vi "GeoData.vi"() -> ()   [LabVIEW 2017] (continued)
PA\tPhiladelphia County\tH6\n19124\t42101\tPhiladelphia\tPA\tPhiladelphia County\tH6\n19152\t42101\tPhiladelphia\tPA\tPhiladelphia County\tH6\n19110\t42101\tPhiladelphia\tPA\tPhiladelphia County\tH6\n19181\t42101\tPhiladelphia\tPA\tPhiladelphia County\tH6\n19119\t42101\tPhiladelphia\tPA\tPhiladelphia County\tH6\n19125\t42101\tPhiladelphia\tPA\tPhiladelphia County\tH6\n19135\t42101\tPhiladelphia\tPA\tPhiladelphia County\tH6\n19140\t42101\tPhiladelphia\tPA\tPhiladelphia County\tH6\n19133\t42101\tPhiladelphia\tPA\tPhiladelphia County\tH6\n19139\t42101\tPhiladelphia\tPA\tPhiladelphia County\tH6\n19134\t42101\tPhiladelphia\tPA\tPhiladelphia County\tH6\n19137\t42101\tPhiladelphia\tPA\tPhiladelphia County\tH6\n19108\t42101\tPhiladelphia\tPA\tPhiladelphia County\tH6\n19190\t42101\tPhiladelphia\tPA\tPhiladelphia County\tH6\n19046\t42101\tJenkintown\tPA\tPhiladelphia County\tH6\n19101\t42101\tPhiladelphia\tPA\tPhiladelphia County\tH6\n19103\t42101\tPhiladelphia\tPA\tPhiladelphia County\tH6\n19123\t42101\tPhiladelphia\tPA\tPhiladelphia County\tH6\n19148\t42101\tPhiladelphia\tPA\tPhiladelphia County\tH6\n19143\t42101\tPhiladelphia\tPA\tPhiladelphia County\tH6\n19150\t42101\tPhiladelphia\tPA\tPhiladelphia County\tH6\n19095\t42101\tWyncote\tPA\tPhiladelphia County\tH6\n19128\t42101\tPhiladelphia\tPA\tPhiladelphia County\tH6\n19131\t42101\tPhiladelphia\tPA\tPhiladelphia County\tH6\n19138\t42101\tPhiladelphia\tPA\tPhiladelphia County\tH6\n19130\t42101\tPhiladelphia\tPA\tPhiladelphia County\tH6\n19144\t42101\tPhiladelphia\tPA\tPhiladelphia County\tH6\n19149\t42101\tPhiladelphia\tPA\tPhiladelphia County\tH6\n19145\t42101\tPhiladelphia\tPA\tPhiladelphia County\tH6\n19176\t42101\tPhiladelphia\tPA\tPhiladelphia County\tH6\n19183\t42101\tPhiladelphia\tPA\tPhiladelphia County\tH6\n19104\t42101\tPhiladelphia\tPA\tPhiladelphia County\tH6\n19112\t42101\tPhiladelphia\tPA\tPhiladelphia County\tH6\n19121\t42101\tPhiladelphia\tPA\tPhiladelphia County\tH6\n19132\t42101\tPhiladelphia\tPA\tPhiladelphia County\tH6\n19192\t42101\tPhiladelphia\tPA\tPhiladelphia County\tH6\n19102\t42101\tPhiladelphia\tPA\tPhiladelphia County\tH6\n19107\t42101\tPhiladelphia\tPA\tPhiladelphia County\tH6\n19127\t42101\tPhiladelphia\tPA\tPhiladelphia County\tH6\n19120\t42101\tPhiladelphia\tPA\tPhiladelphia County\tH6\n19142\t42101\tPhiladelphia\tPA\tPhiladelphia County\tH6\n19114\t42101\tPhiladelphia\tPA\tPhiladelphia County\tH6\n19106\t42101\tPhiladelphia\tPA\tPhiladelphia County\tH6\n19136\t42101\tPhiladelphia\tPA\tPhiladelphia County\tH6\n19153\t42101\tPhiladelphia\tPA\tPhiladelphia County\tH6\n19154\t42101\tPhiladelphia\tPA\tPhiladelphia County\tH6\n19160\t42101\tPhiladelphia\tPA\tPhiladelphia County\tH6\n19172\t42101\tPhiladelphia\tPA\tPhiladelphia County\tH6\n18337\t42103\tMilford\tPA\tPike County\tH1\n18328\t42103\tDingmans ferry\tPA\tPike County\tH1\n18405\t42103\tBeach lake\tPA\tPike County\tH1\n18464\t42103\tTafton\tPA\tPike County\tH1\n18302\t42103\tEast stroudsburg\tPA\tPike County\tH1\n18445\t42103\tNewfoundland\tPA\tPike County\tH1\n18428\t42103\tHawley\tPA\tPike County\tH1\n18325\t42103\tCanadensis\tPA\tPike County\tH1\n18340\t42103\tMillrift\tPA\tPike County\tH1\n18326\t42103\tCresco\tPA\tPike County\tH1\n18425\t42103\tGreeley\tPA\tPike County\tH1\n18436\t42103\tLake ariel\tPA\tPike County\tH1\n18426\t42103\tGreentown\tPA\tPike County\tH1\n18435\t42103\tLackawaxen\tPA\tPike County\tH1\n18371\t42103\tTamiment\tPA\tPike County\tH1\n18458\t42103\tShohola\tPA\tPike County\tH1\n18457\t42103\tRowland\tPA\tPike County\tH1\n18336\t42103\tMatamoras\tPA\tPike County\tH1\n18451\t42103\tPaupack\tPA\tPike County\tH1\n18324\t42103\tBushkill\tPA\tPike County\tH1\n16941\t42105\tGenesee\tPA\tPotter County\tH1\n16746\t42105\tRoulette\tPA\tPotter County\tH1\n16927\t42105\tHarrison valley\tPA\tPotter County\tH1\n16743\t42105\tPort allegany\tPA\tPotter County\tH1\n16923\t42105\tGenesee\tPA\tPotter County\tH1\n16937\t42105\tMills\tPA\tPotter County\tH1\n16950\t42105\tWestfield\tPA\tPotter County\tH1\n16921\t42105\tGaines\tPA\tPotter County\tH1\n16720\t42105\tAustin\tPA\tPotter County\tH1\n16922\t42105\tGaleton\tPA\tPotter County\tH1\n16748\t42105\tShinglehouse\tPA\tPotter County\tH1\n16915\t42105\tCoudersport\tPA\tPotter County\tH1\n17729\t42105\tCross fork\tPA\tPotter County\tH1\n16948\t42105\tUlysses\tPA\tPotter County\tH1\n16943\t42105\tSabinsville\tPA\tPotter County\tH1\n17959\t42107\tNew philadelphia\tPA\tSchuylkill County\tH1\n18211\t42107\tAndreas\tPA\tSchuylkill County\tH1\n17934\t42107\tGilberton\tPA\tSchuylkill County\tH1\n17951\t42107\tMar lin\tPA\tSchuylkill County\tH1\n18220\t42107\tDelano\tPA\tSchuylkill County\tH1\n17933\t42107\tFriedensburg\tPA\tSchuylkill County\tH1\n19549\t42107\tPort clinton\tPA\tSchuylkill County\tH1\n17980\t42107\tTower city\tPA\tSchuylkill County\tH1\n17929\t42107\tCressona\tPA\tSchuylkill County\tH1\n17976\t42107\tShenandoah\tPA\tSchuylkill County\tH1\n18252\t42107\tTamaqua\tPA\tSchuylkill County\tH1\n17970\t42107\tSaint clair\tPA\tSchuylkill County\tH1\n17983\t42107\tValley view\tPA\tSchuylkill County\tH1\n17978\t42107\tSpring glen\tPA\tSchuylkill County\tH1\n18231\t42107\tKelayres\tPA\tSchuylkill County\tH1\n17901\t42107\tPottsville\tPA\tSchuylkill County\tH1\n17938\t42107\tHegins\tPA\tSchuylkill County\tH1\n17921\t42107\tAshland\tPA\tSchuylkill County\tH1\n17931\t42107\tFrackville\tPA\tSchuylkill County\tH1\n17968\t42107\tSacramento\tPA\tSchuylkill County\tH1\n17974\t42107\tSeltzer\tPA\tSchuylkill County\tH1\n17946\t42107\tLost creek\tPA\tSchuylkill County\tH1\n17979\t42107\tSummit station\tPA\tSchuylkill County\tH1\n17963\t42107\tPine grove\tPA\tSchuylkill County\tH1\n17961\t42107\tOrwigsburg\tPA\tSchuylkill County\tH1\n17935\t42107\tGirardville\tPA\tSchuylkill County\tH1\n18214\t42107\tBarnesville\tPA\tSchuylkill County\tH1\n18240\t42107\tNesquehoning\tPA\tSchuylkill County\tH1\n17964\t42107\tPitman\tPA\tSchuylkill County\tH1\n17967\t42107\tRingtown\tPA\tSchuylkill County\tH1\n18245\t42107\tQuakake\tPA\tSchuylkill County\tH1\n17930\t42107\tCumbola\tPA\tSchuylkill County\tH1\n17972\t42107\tSchuylkill haven\tPA\tSchuylkill County\tH1\n17965\t42107\tPort carbon\tPA\tSchuylkill County\tH1\n17948\t42107\tMahanoy city\tPA\tSchuylkill County\tH1\n17953\t42107\tMiddleport\tPA\tSchuylkill County\tH1\n17943\t42107\tLavelle\tPA\tSchuylkill County\tH1\n17949\t42107\tMahanoy plane\tPA\tSchuylkill County\tH1\n17922\t42107\tAuburn\tPA\tSchuylkill County\tH1\n17957\t42107\tMuir\tPA\tSchuylkill County\tH1\n17982\t42107\tTuscarora\tPA\tSchuylkill County\tH1\n17966\t42107\tRavine\tPA\tSchuylkill County\tH1\n17823\t42107\tDornsife\tPA\tSchuylkill County\tH1\n17954\t42107\tMinersville\tPA\tSchuylkill County\tH1\n17981\t42107\tTremont\tPA\tSchuylkill County\tH1\n17941\t42107\tKlingerstown\tPA\tSchuylkill County\tH1\n17985\t42107\tZion grove\tPA\tSchuylkill County\tH1\n18218\t42107\tCoaldale\tPA\tSchuylkill County\tH1\n18202\t42107\tHazleton\tPA\tSchuylkill County\tH1\n17925\t42107\tBrockton\tPA\tSchuylkill County\tH1\n18237\t42107\tMcadoo\tPA\tSchuylkill County\tH1\n17944\t42107\tLlewellyn\tPA\tSchuylkill County\tH1\n17923\t42107\tBranchdale\tPA\tSchuylkill County\tH1\n18242\t42107\tOneida\tPA\tSchuylkill County\tH1\n17960\t42107\tNew ringgold\tPA\tSchuylkill County\tH1\n18241\t42107\tNuremberg\tPA\tSchuylkill County\tH1\n17945\t42107\tLocustdale\tPA\tSchuylkill County\tH1\n17952\t42107\tMary d\tPA\tSchuylkill County\tH1\n17932\t42107\tFrackville\tPA\tSchuylkill County\tH1\n17936\t42107\tGordon\tPA\tSchuylkill County\tH1\n18248\t42107\tSheppton\tPA\tSchuylkill County\tH1\n17843\t42109\tBeaver springs\tPA\tSnyder County\tH1\n17827\t42109\tFreeburg\tPA\tSnyder County\tH1\n17870\t42109\tSelinsgrove\tPA\tSnyder County\tH1\n17086\t42109\tRichfield\tPA\tSnyder County\tH1\n17831\t42109\tHummels wharf\tPA\tSnyder County\tH1\n17841\t42109\tMc clure\tPA\tSnyder County\tH1\n17813\t42109\tBeavertown\tPA\tSnyder County\tH1\n17861\t42109\tPaxtonville\tPA\tSnyder County\tH1\n17833\t42109\tKreamer\tPA\tSnyder County\tH1\n17842\t42109\tMiddleburg\tPA\tSnyder County\tH1\n17864\t42109\tPort trevorton\tPA\tSnyder County\tH1\n17853\t42109\tMount pleasant mills\tPA\tSnyder County\tH1\n17889\t42109\tWinfield\tPA\tSnyder County\tH1\n17862\t42109\tPenns creek\tPA\tSnyder County\tH1\n17882\t42109\tTroxelville\tPA\tSnyder County\tH1\n17876\t42109\tShamokin dam\tPA\tSnyder County\tH1\n17063\t42109\tMilroy\tPA\tSnyder County\tH1\n17844\t42109\tMifflinburg\tPA\tSnyder County\tH1\n17812\t42109\tBeaver springs\tPA\tSnyder County\tH1\n17045\t42109\tLiverpool\tPA\tSnyder County\tH1\n15501\t42111\tSomerset\tPA\tSomerset County\tH1\n15551\t42111\tMarkleton\tPA\tSomerset County\tH1\n15558\t42111\tSalisbury\tPA\tSomerset County\tH1\n15924\t42111\tCairnbrook\tPA\tSomerset County\tH1\n15531\t42111\tBoswell\tPA\tSomerset County\tH1\n15622\t42111\tChampion\tPA\tSomerset County\tH1\n15564\t42111\tWellersburg\tPA\tSomerset County\tH1\n15555\t42111\tQuecreek\tPA\tSomerset County\tH1\n15561\t42111\tSipesville\tPA\tSomerset County\tH1\n15550\t42111\tManns choice\tPA\tSomerset County\tH1\n15545\t42111\tHyndman\tPA\tSomerset County\tH1\n15542\t42111\tGarrett\tPA\tSomerset County\tH1\n15548\t42111\tKantner\tPA\tSomerset County\tH1\n15565\t42111\tWest salisbury\tPA\tSomerset County\tH1\n15532\t42111\tBoynton\tPA\tSomerset County\tH1\n15549\t42111\tListie\tPA\tSomerset County\tH1\n15557\t42111\tRockwood\tPA\tSomerset County\tH1\n15552\t42111\tMeyersdale\tPA\tSomerset County\tH1\n15926\t42111\tCentral city\tPA\tSomerset County\tH1\n15936\t42111\tHooversville\tPA\tSomerset County\tH1\n15937\t42111\tJerome\tPA\tSomerset County\tH1\n15538\t42111\tFairhope\tPA\tSomerset County\tH1\n15935\t42111\tHollsopple\tPA\tSomerset County\tH1\n15510\t42111\tSomerset\tPA\tSomerset County\tH1\n15560\t42111\tShanksville\tPA\tSomerset County\tH1\n15547\t42111\tJennerstown\tPA\tSomerset County\tH1\n15544\t42111\tGray\tPA\tSomerset County\tH1\n15563\t42111\tStoystown\tPA\tSomerset County\tH1\n15562\t42111\tSprings\tPA\tSomerset County\tH1\n15963\t42111\tWindber\tPA\tSomerset County\tH1\n15953\t42111\tSeanor\tPA\tSomerset County\tH1\n15553\t42111\tNew baltimore\tPA\tSomerset County\tH1\n15411\t42111\tAddison\tPA\tSomerset County\tH1\n15530\t42111\tBerlin\tPA\tSomerset County\tH1\n15541\t42111\tFriedens\tPA\tSomerset County\tH1\n15928\t42111\tDavidsville\tPA\tSomerset County\tH1\n15540\t42111\tFort hill\tPA\tSomerset County\tH1\n15559\t42111\tSchellsburg\tPA\tSomerset County\tH1\n15520\t42111\tAcosta\tPA\tSomerset County\tH1\n15485\t42111\tUrsina\tPA\tSomerset County\tH1\n15424\t42111\tConfluence\tPA\tSomerset County\tH1\n15905\t42111\tJohnstown\tPA\tSomerset County\tH1\n15546\t42111\tJenners\tPA\tSomerset County\tH1\n15534\t42111\tBuffalo mills\tPA\tSomerset County\tH1\n15502\t42111\tHidden valley\tPA\tSomerset County\tH1\n18629\t42113\tMehoopany\tPA\tSullivan County\tH1\n18616\t42113\tForksville\tPA\tSullivan County\tH1\n18619\t42113\tHillsgrove\tPA\tSullivan County\tH1\n17814\t42113\tBenton\tPA\tSullivan County\tH1\n18833\t42113\tNew albany\tPA\tSullivan County\tH1\n17758\t42113\tMuncy valley\tPA\tSullivan County\tH1\n17731\t42113\tEagles mere\tPA\tSullivan County\tH1\n17701\t42113\tWilliamsport\tPA\tSullivan County\tH1\n17737\t42113\tHughesville\tPA\tSullivan County\tH1\n18626\t42113\tLaporte\tPA\tSullivan County\tH1\n18628\t42113\tLopez\tPA\tSullivan County\tH1\n18632\t42113\tMildred\tPA\tSullivan County\tH1\n18614\t42113\tDushore\tPA\tSullivan County\tH1\n17768\t42113\tShunk\tPA\tSullivan County\tH1\n18446\t42115\tNicholson\tPA\tSusquehanna County\tH1\n18844\t42115\tSpringville\tPA\tSusquehanna County\tH1\n18823\t42115\tHarford\tPA\tSusquehanna County\tH1\n18842\t42115\tSouth gibson\tPA\tSusquehanna County\tH1\n18828\t42115\tLawton\tPA\tSusquehanna County\tH1\n18801\t42115\tMontrose\tPA\tSusquehanna County\tH1\n18413\t42115\tClifford\tPA\tSusquehanna County\tH1\n18816\t42115\tDimock\tPA\tSusquehanna County\tH1\n18421\t42115\tForest city\tPA\tSusquehanna County\tH1\n18623\t42115\tLaceyville\tPA\tSusquehanna County\tH1\n18830\t42115\tLittle meadows\tPA\tSusquehanna County\tH1\n18430\t42115\tHerrick center\tPA\tSusquehanna County\tH1\n18813\t42115\tBrooklyn\tPA\tSusquehanna County\tH1\n18824\t42115\tHop bottom\tPA\tSusquehanna County\tH1\n18826\t42115\tKingsley\tPA\tSusquehanna County\tH1\n18812\t42115\tBrackney\tPA\tSusquehanna County\tH1\n18441\t42115\tLenoxville\tPA\tSusquehanna County\tH1\n18822\t42115\tHallstead\tPA\tSusquehanna County\tH1\n18821\t42115\tGreat bend\tPA\tSusquehanna County\tH1\n18825\t42115\tJackson\tPA\tSusquehanna County\tH1\n18820\t42115\tGibson\tPA\tSusquehanna County\tH1\n18827\t42115\tLanesboro\tPA\tSusquehanna County\tH1\n18419\t42115\tFactoryville\tPA\tSusquehanna County\tH1\n18462\t42115\tStarrucca\tPA\tSusquehanna County\tH1\n18470\t42115\tUnion dale\tPA\tSusquehanna County\tH1\n18853\t42115\tWyalusing\tPA\tSusquehanna County\tH1\n18465\t42115\tThompson\tPA\tSusquehanna County\tH1\n18818\t42115\tFriendsville\tPA\tSusquehanna County\tH1\n18834\t42115\tNew milford\tPA\tSusquehanna County\tH1\n18407\t42115\tCarbondale\tPA\tSusquehanna County\tH1\n18630\t42115\tMeshoppen\tPA\tSusquehanna County\tH1\n18847\t42115\tSusquehanna\tPA\tSusquehanna County\tH1\n18843\t42115\tSouth montrose\tPA\tSusquehanna County\tH1\n16912\t42117\tBlossburg\tPA\tTioga County\tH1\n16930\t42117\tLiberty\tPA\tTioga County\tH1\n16911\t42117\tArnot\tPA\tTioga County\tH1\n16914\t42117\tColumbia cross roads\tPA\tTioga County\tH1\n16927\t42117\tHarrison valley\tPA\tTioga County\tH1\n16932\t42117\tMainesburg\tPA\tTioga County\tH1\n16929\t42117\tLawrenceville\tPA\tTioga County\tH1\n16933\t42117\tMansfield\tPA\tTioga County\tH1\n16935\t42117\tMiddlebury center\tPA\tTioga County\tH1\n17765\t42117\tRoaring branch\tPA\tTioga County\tH1\n16917\t42117\tCovington\tPA\tTioga County\tH1\n16939\t42117\tMorris run\tPA\tTioga County\tH1\n16946\t42117\tTioga\tPA\tTioga County\tH1\n16950\t42117\tWestfield\tPA\tTioga County\tH1\n16921\t42117\tGaines\tPA\tTioga County\tH1\n16901\t42117\tWellsboro\tPA\tTioga County\tH1\n16928\t42117\tKnoxville\tPA\tTioga County\tH1\n17727\t42117\tCedar run\tPA\tTioga County\tH1\n16922\t42117\tGaleton\tPA\tTioga County\tH1\n16938\t42117\tMorris\tPA\tTioga County\tH1\n17724\t42117\tCanton\tPA\tTioga County\tH1\n16936\t42117\tMillerton\tPA\tTioga County\tH1\n16947\t42117\tTroy\tPA\tTioga County\tH1\n16942\t42117\tOsceola\tPA\tTioga County\tH1\n16920\t42117\tElkland\tPA\tTioga County\tH1\n16943\t42117\tSabinsville\tPA\tTioga County\tH1\n16940\t42117\tNelson\tPA\tTioga County\tH1\n17870\t42119\tSelinsgrove\tPA\tUnion County\tH1\n17845\t42119\tMillmont\tPA\tUnion County\tH1\n17885\t42119\tWeikert\tPA\tUnion County\tH1\n17837\t42119\tLewisburg\tPA\tUnion County\tH1\n17841\t42119\tMc clure\tPA\tUnion County\tH1\n17886\t42119\tWest milton\tPA\tUnion County\tH1\n17835\t42119\tLaurelton\tPA\tUnion County\tH1\n17889\t42119\tWinfield\tPA\tUnion County\tH1\n17855\t42119\tNew berlin\tPA\tUnion County\tH1\n17810\t42119\tAllenwood\tPA\tUnion County\tH1\n17844\t42119\tMifflinburg\tPA\tUnion County\tH1\n17856\t42119\tNew columbia\tPA\tUnion County\tH1\n17829\t42119\tHartleton\tPA\tUnion County\tH1\n17887\t42119\tWhite deer\tPA\tUnion County\tH1\n17880\t42119\tSwengel\tPA\tUnion County\tH1\n16127\t42121\tGrove city\tPA\tVenango County\tH1\n16319\t42121\tCranberry\tPA\tVenango County\tH1\n16364\t42121\tVenus\tPA\tVenango County\tH1\n16314\t42121\tCochranton\tPA\tVenango County\tH1\n16232\t42121\tKnox\tPA\tVenango County\tH1\n16346\t42121\tSeneca\tPA\tVenango County\tH1\n16038\t42121\tHarrisville\tPA\tVenango County\tH1\n16311\t42121\tCarlton\tPA\tVenango County\tH1\n16341\t42121\tPleasantville\tPA\tVenango County\tH1\n16353\t42121\tTionesta\tPA\tVenango County\tH1\n16372\t42121\tClintonville\tPA\tVenango County\tH1\n16373\t42121\tEmlenton\tPA\tVenango County\tH1\n16343\t42121\tReno\tPA\tVenango County\tH1\n16354\t42121\tTitusville\tPA\tVenango County\tH1\n16344\t42121\tRouseville\tPA\tVenango County\tH1\n16317\t42121\tCooperstown\tPA\tVenango County\tH1\n16327\t42121\tGuys mills\tPA\tVenango County\tH1\n16374\t42121\tKennerdell\tPA\tVenango County\tH1\n16301\t42121\tOil city\tPA\tVenango County\tH1\n16362\t42121\tUtica\tPA\tVenango County\tH1\n16153\t42121\tStoneboro\tPA\tVenango County\tH1\n16323\t42121\tFranklin\tPA\tVenango County\tH1\n16342\t42121\tPolk\tPA\tVenango County\tH1\n16313\t42123\tClarendon\tPA\tWarren County\tH1\n16329\t42123\tIrvine\tPA\tWarren County\tH1\n16369\t42123\tWarren\tPA\tWarren County\tH1\n16402\t42123\tBear lake\tPA\tWarren County\tH1\n16352\t42123\tTiona\tPA\tWarren County\tH1\n16407\t42123\tCorry\tPA\tWarren County\tH1\n16436\t42123\tSpring creek\tPA\tWarren County\tH1\n16405\t42123\tColumbus\tPA\tWarren County\tH1\n16368\t42123\tWarren\tPA\tWarren County\tH1\n16367\t42123\tWarren\tPA\tWarren County\tH1\n16416\t42123\tGarland\tPA\tWarren County\tH1\n16354\t42123\tTitusville\tPA\tWarren County\tH1\n16345\t42123\tRussell\tPA\tWarren County\tH1\n16365\t42123\tWarren\tPA\tWarren County\tH1\n16351\t42123\tTidioute\tPA\tWarren County\tH1\n16371\t42123\tYoungsville\tPA\tWarren County\tH1\n16350\t42123\tSugar grove\tPA\tWarren County\tH1\n16347\t42123\tSheffield\tPA\tWarren County\tH1\n16434\t42123\tSpartansburg\tPA\tWarren County\tH1\n16366\t42123\tWarren\tPA\tWarren County\tH1\n16312\t42123\tChandlers valley\tPA\tWarren County\tH1\n16340\t42123\tPittsfield\tPA\tWarren County\tH1\n16420\t42123\tGrand valley\tPA\tWarren County\tH1\n15301\t42125\tWashington\tPA\tWashington County\tH1\n15333\t42125\tFredericktown\tPA\tWashington County\tH1\n15419\t42125\tCalifornia\tPA\tWashington County\tH1\n15019\t42125\tBulger\tPA\tWashington County\tH1\n15363\t42125\tStrabane\tPA\tWashington County\tH1\n15339\t42125\tHendersonville\tPA\tWashington County\tH1\n15368\t42125\tVestaburg\tPA\tWashington County\tH1\n15434\t42125\tElco\tPA\tWashington County\tH1\n15012\t42125\tBelle vernon\tPA\tWashington County\tH1\n15022\t42125\tCharleroi\tPA\tWashington County\tH1\n16102\t42125\tNew castle\tPA\tWashington County\tH1\n15060\t42125\tMidway\tPA\tWashington County\tH1\n15321\t42125\tCecil\tPA\tWashington County\tH1\n15432\t42125\tDunlevy\tPA\tWashington County\tH1\n15378\t42125\tWestland\tPA\tWashington County\tH1\n15004\t42125\tAtlasburg\tPA\tWashington County\tH1\n15331\t42125\tEllsworth\tPA\tWashington County\tH1\n15017\t42125\tBridgeville\tPA\tWashington County\tH1\n15026\t42125\tClinton\tPA\tWashington County\tH1\n15360\t42125\tScenery hill\tPA\tWashington County\tH1\n15345\t42125\tMarianna\tPA\tWashington County\tH1\n15348\t42125\tMillsboro\tPA\tWashington County\tH1\n15365\t42125\tTaylorstown\tPA\tWashington County\tH1\n15021\t42125\tBurgettstown\tPA\tWashington County\tH1\n15054\t42125\tLangeloth\tPA\tWashington County\tH1\n15102\t42125\tBethel park\tPA\tWashington County\tH1\n15129\t42125\tSouth park\tPA\tWashington County\tH1\n15126\t42125\tImperial\tPA\tWashington County\tH1\n15332\t42125\tFinleyville\tPA\tWashington County\tH1\n15427\t42125\tDaisytown\tPA\tWashington County\tH1\n15340\t42125\tHickory\tPA\tWashington County\tH1\n15477\t42125\tRoscoe\tPA\tWashington County\tH1\n15313\t42125\tBeallsville\tPA\tWashington County\tH1\n15358\t42125\tRicheyville\tPA\tWashington County\tH1\n15379\t42125\tWest middletown\tPA\tWashington County\tH1\n15336\t42125\tGastonville\tPA\tWashington County\tH1\n15314\t42125\tBentleyville\tPA\tWashington County\tH1\n15317\t42125\tCanonsburg\tPA\tWashington County\tH1\n15311\t42125\tAmity\tPA\tWashington County\tH1\n15312\t42125\tAvella\tPA\tWashington County\tH1\n15417\t42125\tBrownsville\tPA\tWashington County\tH1\n15367\t42125\tVenetia\tPA\tWashington County\tH1\n15053\t42125\tJoffre\tPA\tWashington County\tH1\n15330\t42125\tEighty four\tPA\tWashington County\tH1\n15361\t42125\tSouthview\tPA\tWashington County\tH1\n15078\t42125\tSlovan\tPA\tWashington County\tH1\n15067\t42125\tNew eagle\tPA\tWashington County\tH1\n15033\t42125\tDonora\tPA\tWashington County\tH1\n15057\t42125\tMc donald\tPA\tWashington County\tH1\n15241\t42125\tPittsburgh\tPA\tWashington County\tH1\n15329\t42125\tProsperity\tPA\tWashington County\tH1\n15370\t42125\tWaynesburg\tPA\tWashington County\tH1\n15377\t42125\tWest finley\tPA\tWashington County\tH1\n15324\t42125\tCokeburg\tPA\tWashington County\tH1\n15366\t42125\tVan voorhis\tPA\tWashington County\tH1\n15342\t42125\tHouston\tPA\tWashington County\tH1\n15323\t42125\tClaysville\tPA\tWashington County\tH1\n15423\t42125\tCoal center\tPA\tWashington County\tH1\n15055\t42125\tLawrence\tPA\tWashington County\tH1\n15429\t42125\tDenbo\tPA\tWashington County\tH1\n15483\t42125\tStockdale\tPA\tWashington County\tH1\n15350\t42125\tMuse\tPA\tWashington County\tH1\n15412\t42125\tAllenport\tPA\tWashington County\tH1\n15063\t42125\tMonongahela\tPA\tWashington County\tH1\n15376\t42125\tWest alexander\tPA\tWashington County\tH1\n15322\t42125\tClarksville\tPA\tWashington County\tH1\n15357\t42125\tRices landing\tPA\tWashington County\tH1\n15347\t42125\tMeadow lands\tPA\tWashington County\tH1\n18405\t42127\tBeach lake\tPA\tWayne County\tH1\n18415\t42127\tDamascus\tPA\tWayne County\tH1\n18427\t42127\tHamlin\tPA\tWayne County\tH1\n18449\t42127\tOrson\tPA\tWayne County\tH1\n18444\t42127\tMoscow\tPA\tWayne County\tH1\n18461\t42127\tStarlight\tPA\tWayne County\tH1\n18438\t42127\tLakeville\tPA\tWayne County\tH1\n18456\t42127\tPrompton\tPA\tWayne County\tH1\n18421\t42127\tForest city\tPA\tWayne County\tH1\n18445\t42127\tNewfoundland\tPA\tWayne County\tH1\n18428\t42127\tHawley\tPA\tWayne County\tH1\n18460\t42127\tSouth sterling\tPA\tWayne County\tH1\n18430\t42127\tHerrick center\tPA\tWayne County\tH1\n18436\t42127\tLake ariel\tPA\tWayne County\tH1\n18439\t42127\tLakewood\tPA\tWayne County\tH1\n18426\t42127\tGreentown\tPA\tWayne County\tH1\n18466\t42127\tTobyhanna\tPA\tWayne County\tH1\n18472\t42127\tWaymart\tPA\tWayne County\tH1\n18473\t42127\tWhite mills\tPA\tWayne County\tH1\n18431\t42127\tHonesdale\tPA\tWayne County\tH1\n18417\t42127\tEquinunk\tPA\tWayne County\tH1\n18437\t42127\tLake como\tPA\tWayne County\tH1\n18469\t42127\tTyler hill\tPA\tWayne County\tH1\n18434\t42127\tJessup\tPA\tWayne County\tH1\n18459\t42127\tSouth canaan\tPA\tWayne County\tH1\n18462\t42127\tStarrucca\tPA\tWayne County\tH1\n18470\t42127\tUnion dale\tPA\tWayne County\tH1\n18443\t42127\tMilanville\tPA\tWayne County\tH1\n18463\t42127\tSterling\tPA\tWayne County\tH1\n18465\t42127\tThompson\tPA\tWayne County\tH1\n18455\t42127\tPreston park\tPA\tWayne County\tH1\n18454\t42127\tPoyntelle\tPA\tWayne County\tH1\n18424\t42127\tGouldsboro\tPA\tWayne County\tH1\n18847\t42127\tSusquehanna\tPA\tWayne County\tH1\n18453\t42127\tPleasant mount\tPA\tWayne County\tH1\n15501\t42129\tSomerset\tPA\tWestmoreland County\tH1\n15627\t42129\tDerry\tPA\tWestmoreland County\tH1\n15636\t42129\tHarrison city\tPA\tWestmoreland County\tH1\n15690\t42129\tVandergrift\tPA\tWestmoreland County\tH1\n15923\t42129\tBolivar\tPA\tWestmoreland County\tH1\n15531\t42129\tBoswell\tPA\tWestmoreland County\tH1\n15626\t42129\tDelmont\tPA\tWestmoreland County\tH1\n15660\t42129\tLowber\tPA\tWestmoreland County\tH1\n15622\t42129\tChampion\tPA\tWestmoreland County\tH1\n15646\t42129\tJones mills\tPA\tWestmoreland County\tH1\n15641\t42129\tHyde park\tPA\tWestmoreland County\tH1\n15698\t42129\tYukon\tPA\tWestmoreland County\tH1\n15691\t42129\tWendel\tPA\tWestmoreland County\tH1\n15662\t42129\tLuxor\tPA\tWestmoreland County\tH1\n15012\t42129\tBelle vernon\tPA\tWestmoreland County\tH1\n15062\t42129\tMonessen\tPA\tWestmoreland County\tH1\n15137\t42129\tNorth versailles\tPA\tWestmoreland County\tH1\n15479\t42129\tSmithton\tPA\tWestmoreland County\tH1\n15601\t42129\tGreensburg\tPA\tWestmoreland County\tH1\n15642\t42129\tIrwin\tPA\tWestmoreland County\tH1\n15656\t42129\tLeechburg\tPA\tWestmoreland County\tH1\n15613\t42129\tApollo\tPA\tWestmoreland County\tH1\n15637\t42129\tHerminie\tPA\tWestmoreland County\tH1\n15665\t42129\tManor\tPA\tWestmoreland County\tH1\n15687\t42129\tStahlstown\tPA\tWestmoreland County\tH1\n15087\t42129\tWebster\tPA\tWestmoreland County\tH1\n15611\t42129\tAdamsburg\tPA\tWestmoreland County\tH1\n15633\t42129\tForbes road\tPA\tWestmoreland County\tH1\n15647\t42129\tLarimer\tPA\tWestmoreland County\tH1\n15629\t42129\tEast vandergrift\tPA\tWestmoreland County\tH1\n15448\t42129\tJacobs creek\tPA\tWestmoreland County\tH1\n15624\t42129\tCrabtree\tPA\tWestmoreland County\tH1\n15239\t42129\tPittsburgh\tPA\tWestmoreland County\tH1\n15650\t42129\tLatrobe\tPA\tWestmoreland County\tH1\n15677\t42129\tRector\tPA\tWestmoreland County\tH1\n15675\t42129\tPenn\tPA\tWestmoreland County\tH1\n15612\t42129\tAlverton\tPA\tWestmoreland County\tH1\n15619\t42129\tBovard\tPA\tWestmoreland County\tH1\n15779\t42129\tTorrance\tPA\tWestmoreland County\tH1\n15638\t42129\tHostetter\tPA\tWestmoreland County\tH1\n15639\t42129\tHunker\tPA\tWestmoreland County\tH1\n15618\t42129\tAvonmore\tPA\tWestmoreland County\tH1\n15680\t42129\tSalina\tPA\tWestmoreland County\tH1\n15606\t42129\tGreensburg\tPA\tWestmoreland County\tH1\n15068\t42129\tNew kensington\tPA\tWestmoreland County\tH1\n15089\t42129\tWest newton\tPA\tWestmoreland County\tH1\n15083\t42129\tSutersville\tPA\tWestmoreland County\tH1\n15632\t42129\tExport\tPA\tWestmoreland County\tH1\n15610\t42129\tAcme\tPA\tWestmoreland County\tH1\n15671\t42129\tNew derry\tPA\tWestmoreland County\tH1\n15668\t42129\tMurrysville\tPA\tWestmoreland County\tH1\n15695\t42129\tWyano\tPA\tWestmoreland County\tH1\n15697\t42129\tYoungwood\tPA\tWestmoreland County\tH1\n15628\t42129\tDonegal\tPA\tWestmoreland County\tH1\n15684\t42129\tSlickville\tPA\tWestmoreland County\tH1\n15696\t42129\tYoungstown\tPA\tWestmoreland County\tH1\n15663\t42129\tMadison\tPA\tWestmoreland County\tH1\n15069\t42129\tNew kensington\tPA\tWestmoreland County\tH1\n15146\t42129\tMonroeville\tPA\tWestmoreland County\tH1\n15131\t42129\tMckeesport\tPA\tWestmoreland County\tH1\n15658\t42129\tLigonier\tPA\tWestmoreland County\tH1\n15670\t42129\tNew alexandria\tPA\tWestmoreland County\tH1\n15679\t42129\tRuffs dale\tPA\tWestmoreland County\tH1\n15688\t42129\tTarrs\tPA\tWestmoreland County\tH1\n15615\t42129\tArdara\tPA\tWestmoreland County\tH1\n15616\t42129\tArmbrust\tPA\tWestmoreland County\tH1\n15621\t42129\tCalumet\tPA\tWestmoreland County\tH1\n15664\t42129\tMammoth\tPA\tWestmoreland County\tH1\n15617\t42129\tArona\tPA\tWestmoreland County\tH1\n15644\t42129\tJeannette\tPA\tWestmoreland County\tH1\n15666\t42129\tMount pleasant\tPA\tWestmoreland County\tH1\n15672\t42129\tNew stanton\tPA\tWestmoreland County\tH1\n15683\t42129\tScottdale\tPA\tWestmoreland County\tH1\n15717\t42129\tBlairsville\tPA\tWestmoreland County\tH1\n15661\t42129\tLoyalhanna\tPA\tWestmoreland County\tH1\n15681\t42129\tSaltsburg\tPA\tWestmoreland County\tH1\n15678\t42129\tRillton\tPA\tWestmoreland County\tH1\n15954\t42129\tSeward\tPA\tWestmoreland County\tH1\n15620\t42129\tBradenville\tPA\tWestmoreland County\tH1\n15692\t42129\tWestmoreland city\tPA\tWestmoreland County\tH1\n15640\t42129\tHutchinson\tPA\tWestmoreland County\tH1\n15072\t42129\tPricedale\tPA\tWestmoreland County\tH1\n15625\t42129\tDarragh\tPA\tWestmoreland County\tH1\n15693\t42129\tWhitney\tPA\tWestmoreland County\tH1\n15689\t42129\tUnited\tPA\tWestmoreland County\tH1\n15085\t42129\tTrafford\tPA\tWestmoreland County\tH1\n15655\t42129\tLaughlintown\tPA\tWestmoreland County\tH1\n15634\t42129\tGrapeville\tPA\tWestmoreland County\tH1\n15944\t42129\tNew florence\tPA\tWestmoreland County\tH1\n16229\t42129\tFreeport\tPA\tWestmoreland County\tH1\n15623\t42129\tClaridge\tPA\tWestmoreland County\tH1\n15676\t42129\tPleasant unity\tPA\tWestmoreland County\tH1\n15685\t42129\tSouthwest\tPA\tWestmoreland County\tH1\n15635\t42129\tHannastown\tPA\tWestmoreland County\tH1\n15674\t42129\tNorvelt\tPA\tWestmoreland County\tH1\n18446\t42131\tNicholson\tPA\tWyoming County\tH1\n18629\t42131\tMehoopany\tPA\tWyoming County\tH1\n18844\t42131\tSpringville\tPA\tWyoming County\tH1\n18414\t42131\tDalton\tPA\tWyoming County\tH1\n18623\t42131\tLaceyville\tPA\tWyoming County\tH1\n18618\t42131\tHarveys lake\tPA\tWyoming County\tH1\n18419\t42131\tFactoryville\tPA\tWyoming County\tH1\n18657\t42131\tTunkhannock\tPA\tWyoming County\tH1\n18625\t42131\tLake winola\tPA\tWyoming County\tH1\n18636\t42131\tNoxen\tPA\tWyoming County\tH1\n18615\t42131\tFalls\tPA\tWyoming County\tH1\n18614\t42131\tDushore\tPA\tWyoming County\tH1\n18612\t42131\tDallas\tPA\tWyoming County\tH1\n18630\t42131\tMeshoppen\tPA\tWyoming County\tH1\n17403\t42133\tYork\tPA\tYork County\tH1\n17406\t42133\tYork\tPA\tYork County\tH1\n17407\t42133\tYork\tPA\tYork County\tH1\n17368\t42133\tWrightsville\tPA\tYork County\tH1\n17301\t42133\tAbbottstown\tPA\tYork County\tH1\n17404\t42133\tYork\tPA\tYork County\tH1\n17362\t42133\tSpring grove\tPA\tYork County\tH1\n17363\t42133\tStewartstown\tPA\tYork County\tH1\n17405\t42133\tYork\tPA\tYork County\tH1\n17370\t42133\tYork haven\tPA\tYork County\tH1\n17364\t42133\tThomasville\tPA\tYork County\tH1\n17315\t42133\tDover\tPA\tYork County\tH1\n17331\t42133\tHanover\tPA\tYork County\tH1\n17352\t42133\tNew park\tPA\tYork County\tH1\n17317\t42133\tEast prospect\tPA\tYork County\tH1\n17311\t42133\tCodorus\tPA\tYork County\tH1\n17332\t42133\tHanover\tPA\tYork County\tH1\n17309\t42133\tBrogue\tPA\tYork County\tH1\n17316\t42133\tEast berlin\tPA\tYork County\tH1\n17322\t42133\tFelton\tPA\tYork County\tH1\n17329\t42133\tGlenville\tPA\tYork County\tH1\n17360\t42133\tSeven valleys\tPA\tYork County\tH1\n17401\t42133\tYork\tPA\tYork County\tH1\n17402\t42133\tYork\tPA\tYork County\tH1\n17355\t42133\tRailroad\tPA\tYork County\tH1\n17312\t42133\tCraley\tPA\tYork County\tH1\n17345\t42133\tManchester\tPA\tYork County\tH1\n17323\t42133\tFranklintown\tPA\tYork County\tH1\n17371\t42133\tYork new salem\tPA\tYork County\tH1\n17019\t42133\tDillsburg\tPA\tYork County\tH1\n17313\t42133\tDallastown\tPA\tYork County\tH1\n17318\t42133\tEmigsville\tPA\tYork County\tH1\n17347\t42133\tMount wolf\tPA\tYork County\tH1\n17408\t42133\tYork\tPA\tYork County\tH1\n17361\t42133\tShrewsbury\tPA\tYork County\tH1\n17365\t42133\tWellsville\tPA\tYork County\tH1\n17011\t42133\tCamp hill\tPA\tYork County\tH1\n17070\t42133\tNew cumberland\tPA\tYork County\tH1\n17319\t42133\tEtters\tPA\tYork County\tH1\n17302\t42133\tAirville\tPA\tYork County\tH1\n17349\t42133\tNew freedom\tPA\tYork County\tH1\n17356\t42133\tRed lion\tPA\tYork County\tH1\n17366\t42133\tWindsor\tPA\tYork County\tH1\n17372\t42133\tYork springs\tPA\tYork County\tH1\n17342\t42133\tLoganville\tPA\tYork County\tH1\n17358\t42133\tRossville\tPA\tYork County\tH1\n17055\t42133\tMechanicsburg\tPA\tYork County\tH1\n17314\t42133\tDelta\tPA\tYork County\tH1\n17327\t42133\tGlen rock\tPA\tYork County\tH1\n17339\t42133\tLewisberry\tPA\tYork County\tH1\n17321\t42133\tFawn grove\tPA\tYork County\tH1\n2806\t44001\tBarrington\tRI\tBristol County\tH4\n2809\t44001\tBristol\tRI\tBristol County\tH4\n2885\t44001\tWarren\tRI\tBristol County\tH4\n2915\t44001\tRiverside\tRI\tBristol County\tH4\n2887\t44003\tWarwick\tRI\tKent County\tH4\n2818\t44003\tEast greenwich\tRI\tKent County\tH4\n2893\t44003\tWest warwick\tRI\tKent County\tH4\n2888\t44003\tWarwick\tRI\tKent County\tH4\n2889\t44003\tWarwick\tRI\tKent County\tH4\n2852\t44003\tNorth kingstown\tRI\tKent County\tH4\n2827\t44003\tGreene\tRI\tKent County\tH4\n2831\t44003\tHope\tRI\tKent County\tH4\n2817\t44003\tWest greenwich\tRI\tKent County\tH4\n2886\t44003\tWarwick\tRI\tKent County\tH4\n2920\t44003\tCranston\tRI\tKent County\tH4\n2816\t44003\tCoventry\tRI\tKent County\tH4\n2822\t44003\tExeter\tRI\tKent County\tH4\n2825\t44003\tFoster\tRI\tKent County\tH4\n2801\t44005\tAdamsville\tRI\tNewport County\tH4\n2878\t44005\tTiverton\tRI\tNewport County\tH4\n2841\t44005\tNewport\tRI\tNewport County\tH4\n2842\t44005\tMiddletown\tRI\tNewport County\tH4\n2837\t44005\tLittle compton\tRI\tNewport County\tH4\n2871\t44005\tPortsmouth\tRI\tNewport County\tH4\n2840\t44005\tNewport\tRI\tNewport County\tH4\n2872\t44005\tPrudence island\tRI\tNewport County\tH4\n2835\t44005\tJamestown\tRI\tNewport County\tH4\n2828\t44007\tGreenville\tRI\tProvidence County\tH4\n2823\t44007\tFiskeville\tRI\tProvidence County\tH4\n2918\t44007\tProvidence\tRI\tProvidence County\tH4\n2838\t44007\tManville\tRI\tProvidence County\tH4\n2859\t44007\tPascoag\tRI\tProvidence County\tH4\n2909\t44007\tProvidence\tRI\tProvidence County\tH4\n2914\t44007\tEast providence\tRI\tProvidence County\tH4\n2912\t44007\tProvidence\tRI\tProvidence County\tH4\n2908\t44007\tProvidence\tRI\tProvidence County\tH4\n2905\t44007\tProvidence\tRI\tProvidence County\tH4\n2815\t44007\tClayville\tRI\tProvidence County\tH4\n2903\t44007\tProvidence\tRI\tProvidence County\tH4\n2896\t44007\tNorth smithfield\tRI\tProvidence County\tH4\n2830\t44007\tHarrisville\tRI\tProvidence County\tH4\n2831\t44007\tHope\tRI\tProvidence County\tH4\n2857\t44007\tNorth scituate\tRI\tProvidence County\tH4\n2895\t44007\tWoonsocket\tRI\tProvidence County\tH4\n2907\t44007\tProvidence\tRI\tProvidence County\tH4\n2802\t44007\tAlbion\tRI\tProvidence County\tH4\n2829\t44007\tHarmony\tRI\tProvidence County\tH4\n2861\t44007\tPawtucket\tRI\tProvidence County\tH4\n2910\t44007\tCranston\tRI\tProvidence County\tH4\n2906\t44007\tProvidence\tRI\tProvidence County\tH4\n2911\t44007\tNorth providence\tRI\tProvidence County\tH4\n2916\t44007\tRumford\tRI\tProvidence County\tH4\n2876\t44007\tSlatersville\tRI\tProvidence County\tH4\n2860\t44007\tPawtucket\tRI\tProvidence County\tH4\n2858\t44007\tOakland\tRI\tProvidence County\tH4\n2863\t44007\tCentral falls\tRI\tProvidence County\tH4\n2904\t44007\tProvidence\tRI\tProvidence County\tH4\n2901\t44007\tProvidence\tRI\tProvidence County\tH4\n2920\t44007\tCranston\tRI\tProvidence County\tH4\n2826\t44007\tGlendale\tRI\tProvidence County\tH4\n2839\t44007\tMapleville\tRI\tProvidence County\tH4\n2824\t44007\tForestdale\tRI\tProvidence County\tH4\n2814\t44007\tChepachet\tRI\tProvidence County\tH4\n2816\t44007\tCoventry\tRI\tProvidence County\tH4\n2825\t44007\tFoster\tRI\tProvidence County\tH4\n2864\t44007\tCumberland\tRI\tProvidence County\tH4\n2865\t44007\tLincoln\tRI\tProvidence County\tH4\n2862\t44007\tPawtucket\tRI\tProvidence County\tH4\n2915\t44007\tRiverside\tRI\tProvidence County\tH4\n2919\t44007\tJohnston\tRI\tProvidence County\tH4\n2917\t44007\tSmithfield\tRI\tProvidence County\tH4\n2921\t44007\tCranston\tRI\tProvidence County\tH4\n2940\t44007\tProvidence\tRI\tProvidence County\tH4\n2902\t44007\tProvidence\tRI\tProvidence County\tH4\n2808\t44009\tBradford\tRI\tWashington County\tH4\n2883\t44009\tPeace dale\tRI\tWashington County\tH4\n2875\t44009\tShannock\tRI\tWashington County\tH4\n2836\t44009\tKenyon\tRI\tWashington County\tH4\n2813\t44009\tCharlestown\tRI\tWashington County\tH4\n2832\t44009\tHope valley\tRI\tWashington County\tH4\n2874\t44009\tSaunderstown\tRI\tWashington County\tH4\n2891\t44009\tWesterly\tRI\tWashington County\tH4\n2873\t44009\tRockville\tRI\tWashington County\tH4\n2833\t44009\tHopkinton\tRI\tWashington County\tH4\n2881\t44009\tKingston\tRI\tWashington County\tH4\n2812\t44009\tCarolina\tRI\tWashington County\tH4\n2804\t44009\tAshaway\tRI\tWashington County\tH4\n2852\t44009\tNorth kingstown\tRI\tWashington County\tH4\n2877\t44009\tSlocum\tRI\tWashington County\tH4\n2882\t44009\tNarragansett\tRI\tWashington County\tH4\n2892\t44009\tWest kingston\tRI\tWashington County\tH4\n2894\t44009\tWood river junction\tRI\tWashington County\tH4\n2898\t44009\tWyoming\tRI\tWashington County\tH4\n2822\t44009\tExeter\tRI\tWashington County\tH4\n2879\t44009\tWakefield\tRI\tWashington County\tH4\n2880\t44009\tWakefield\tRI\tWashington County\tH4\n2807\t44009\tBlock island\tRI\tWashington County\tH4\n29627\t45001\tBelton\tSC\tAbbeville County\tH1\n29620\t45001\tAbbeville\tSC\tAbbeville County\tH1\n29649\t45001\tGreenwood\tSC\tAbbeville County\tH1\n29638\t45001\tDonalds\tSC\tAbbeville County\tH1\n29639\t45001\tDue west\tSC\tAbbeville County\tH1\n29628\t45001\tCalhoun falls\tSC\tAbbeville County\tH1\n29646\t45001\tGreenwood\tSC\tAbbeville County\tH1\n29653\t45001\tHodges\tSC\tAbbeville County\tH1\n29819\t45001\tBradley\tSC\tAbbeville County\tH1\n29659\t45001\tLowndesville\tSC\tAbbeville County\tH1\n29654\t45001\tHonea path\tSC\tAbbeville County\tH1\n29655\t45001\tIva\tSC\tAbbeville County\tH1\n29692\t45001\tWare shoals\tSC\tAbbeville County\tH1\n29801\t45003\tAiken\tSC\tAiken County\tH1\n29841\t45003\tNorth augusta\tSC\tAiken County\tH1\n29129\t45003\tRidge spring\tSC\tAiken County\tH1\n29839\t45003\tMontmorenci\tSC\tAiken County\tH1\n29146\t45003\tSpringfield\tSC\tAiken County\tH1\n29805\t45003\tAiken\tSC\tAiken County\tH1\n29851\t45003\tWarrenville\tSC\tAiken County\tH1\n29853\t45003\tWilliston\tSC\tAiken County\tH1\n29847\t45003\tTrenton\tSC\tAiken County\tH1\n29809\t45003\tNew ellenton\tSC\tAiken County\tH1\n29006\t45003\tBatesburg\tSC\tAiken County\tH1\n29137\t45003\tSalley\tSC\tAiken County\tH1\n29834\t45003\tLangley\tSC\tAiken County\tH1\n29850\t45003\tVaucluse\tSC\tAiken County\tH1\n29856\t45003\tWindsor\tSC\tAiken County\tH1\n29860\t45003\tNorth augusta\tSC\tAiken County\tH1\n29816\t45003\tBath\tSC\tAiken County\tH1\n29164\t45003\tWagener\tSC\tAiken County\tH1\n29803\t45003\tAiken\tSC\tAiken County\tH1\n29831\t45003\tJackson\tSC\tAiken County\tH1\n29832\t45003\tJohnston\tSC\tAiken County\tH1\n29828\t45003\tGloverville\tSC\tAiken County\tH1\n29802\t45003\tAiken\tSC\tAiken County\tH1\n29861\t45003\tNorth augusta\tSC\tAiken County\tH1\n29822\t45003\tClearwater\tSC\tAiken County\tH1\n29105\t45003\tMonetta\tSC\tAiken County\tH1\n29804\t45003\tAiken\tSC\tAiken County\tH1\n29829\t45003\tGraniteville\tSC\tAiken County\tH1\n29842\t45003\tBeech island\tSC\tAiken County\tH1\n29827\t45005\tFairfax\tSC\tAllendale County\tH1\n29932\t45005\tLuray\tSC\tAllendale County\tH1\n29836\t45005\tMartin\tSC\tAllendale County\tH1\n29810\t45005\tAllendale\tSC\tAllendale County\tH1\n29911\t45005\tBrunson\tSC\tAllendale County\tH1\n29812\t45005\tBarnwell\tSC\tAllendale County\tH1\n29849\t45005\tUlmer\tSC\tAllendale County\tH1\n29846\t45005\tSycamore\tSC\tAllendale County\tH1\n29627\t45007\tBelton\tSC\tAnderson County\tH1\n29623\t45007\tAnderson\tSC\tAnderson County\tH1\n29625\t45007\tAnderson\tSC\tAnderson County\tH1\n29611\t45007\tGreenville\tSC\tAnderson County\tH1\n29621\t45007\tAnderson\tSC\tAnderson County\tH1\n29643\t45007\tFair play\tSC\tAnderson County\tH1\n29626\t45007\tAnderson\tSC\tAnderson County\tH1\n29689\t45007\tTownville\tSC\tAnderson County\tH1\n29622\t45007\tAnderson\tSC\tAnderson County\tH1\n29669\t45007\tPelzer\tSC\tAnderson County\tH1\n29630\t45007\tCentral\tSC\tAnderson County\tH1\n29670\t45007\tPendleton\tSC\tAnderson County\tH1\n29656\t45007\tLa france\tSC\tAnderson County\tH1\n29677\t45007\tSandy springs\tSC\tAnderson County\tH1\n29654\t45007\tHonea path\tSC\tAnderson County\tH1\n29684\t45007\tStarr\tSC\tAnderson County\tH1\n29697\t45007\tWilliamston\tSC\tAnderson County\tH1\n29624\t45007\tAnderson\tSC\tAnderson County\tH1\n29631\t45007\tClemson\tSC\tAnderson County\tH1\n29642\t45007\tEasley\tSC\tAnderson County\tH1\n29657\t45007\tLiberty\tSC\tAnderson County\tH1\n29655\t45007\tIva\tSC\tAnderson County\tH1\n29673\t45007\tPiedmont\tSC\tAnderson County\tH1\n29817\t45009\tBlackville\tSC\tBamberg County\tH1\n29003\t45009\tBamberg\tSC\tBamberg County\tH1\n29038\t45009\tCope\tSC\tBamberg County\tH1\n29042\t45009\tDenmark\tSC\tBamberg County\tH1\n29081\t45009\tEhrhardt\tSC\tBamberg County\tH1\n29481\t45009\tSmoaks\tSC\tBamberg County\tH1\n29843\t45009\tOlar\tSC\tBamberg County\tH1\n29082\t45009\tLodge\tSC\tBamberg County\tH1\n29432\t45009\tBranchville\tSC\tBamberg County\tH1\n29817\t45011\tBlackville\tSC\tBarnwell County\tH1\n29836\t45011\tMartin\tSC\tBarnwell County\tH1\n29812\t45011\tBarnwell\tSC\tBarnwell County\tH1\n29853\t45011\tWilliston\tSC\tBarnwell County\tH1\n29849\t45011\tUlmer\tSC\tBarnwell County\tH1\n29813\t45011\tHilda\tSC\tBarnwell County\tH1\n29808\t45011\tAiken\tSC\tBarnwell County\tH1\n29843\t45011\tOlar\tSC\tBarnwell County\tH1\n
